vi "p09.vi"() -> ()   [LabVIEW 2015]
uses:
  <vilib>/regexp/Match Regular Expression.xnode
panel:
  out "Spreadsheet string -> array":dbl[][](array[numeric])
  out "Array -> spreadsheet string":string
  in  "time stamp":timestamp
  out "date/time string":string
  out "Scan - 2":string
  out "Scan -1":string
  out "remaining string":string
  out "X":dbl
  out "Y":i32
  out "Remaining String":string
  out "Unsigned Byte array to String":string
  out "String to Unsigned Byte array":u8[](array[numeric])
  out "String to Path":path
  out "Path to String":string
  out "Array to Path":path
  out "Path to Array":string[](array[string])
  out "offset past match":i32
  out "after match":string
  out "whole match":string
  out "before match":string
  out "offset past replacement":i32
  out "number of replacements":i32
  out "result string":string
  out "replaced substring":string
  out "result string":string
  out "string substring":string
  out "resulting string":string
  out "offset of match":i32
  out "match + rest of string":string
  out "substring before match":string
  out "offset past match":i32
  out "after substring":string
  out "match substring":string
  out "before substring":string
  out "Append String":string
  out "float-10 digit-2 decimal\n\"0\" padding":string
  out "binary-4 digit-\"0\"":string
  out "binary-4 digit-\" \"":string
  out "binary-without padding":string
  out "concatenated string":string
  out "Array":string[](array[string])
  out "CR & LF":string
  out "Double line feed":string
  out "Remainder":i32
  out "Quotient":i32
  out "Quotient":i32[](array[numeric])
  out "Remainder":i32[](array[numeric])
  out "Shift register":dbl[](array[numeric])
  out "Tunnel":dbl[](array[numeric])
  out "Final":dbl[](array[numeric])
  out "not of I16":i16
  out "not of U8":u8
  out "word swapped":i32 format="%032b"
  out "byte swapped":u32 format="%032b"
  out "?":dynamicdata(graph)
  out "number in bool":bool[](array[boolean])
  out "bool in number":dbl[](array[numeric])
  out "bool":bool[](array[boolean])
  out "number":dbl[](array[numeric])
  # "EXAMPLE - 1"
  # "EXAMPLE - 3"
  # "PATH / ARRAY FUNCTION"
  # "EXAMPLE - 2"
  # "APPEND T/F STRING"
  # "REPLACE SUBSTRING"
  # "MATCH REGULAR EXPRESSION"
  # "SCAN FROM STRING"
  # "ARRAY <-> SPREADSHEET\n STRING"
  # "EXAMPLE - 5"
  # "EXAMPLE - 4"
  # "EXAMPLE - 6"
  # "EXAMPLE - 7"
  # "FORMAT INTO STRING"
  # "SEARCH / SPLIT STRING"
  # "STRING SUBSET FUNCTION"
  # "MATCH PATTERN"
  # "STRING SUBSET FUNCTION"
  # "FORMAT DATE/TIME STRING"
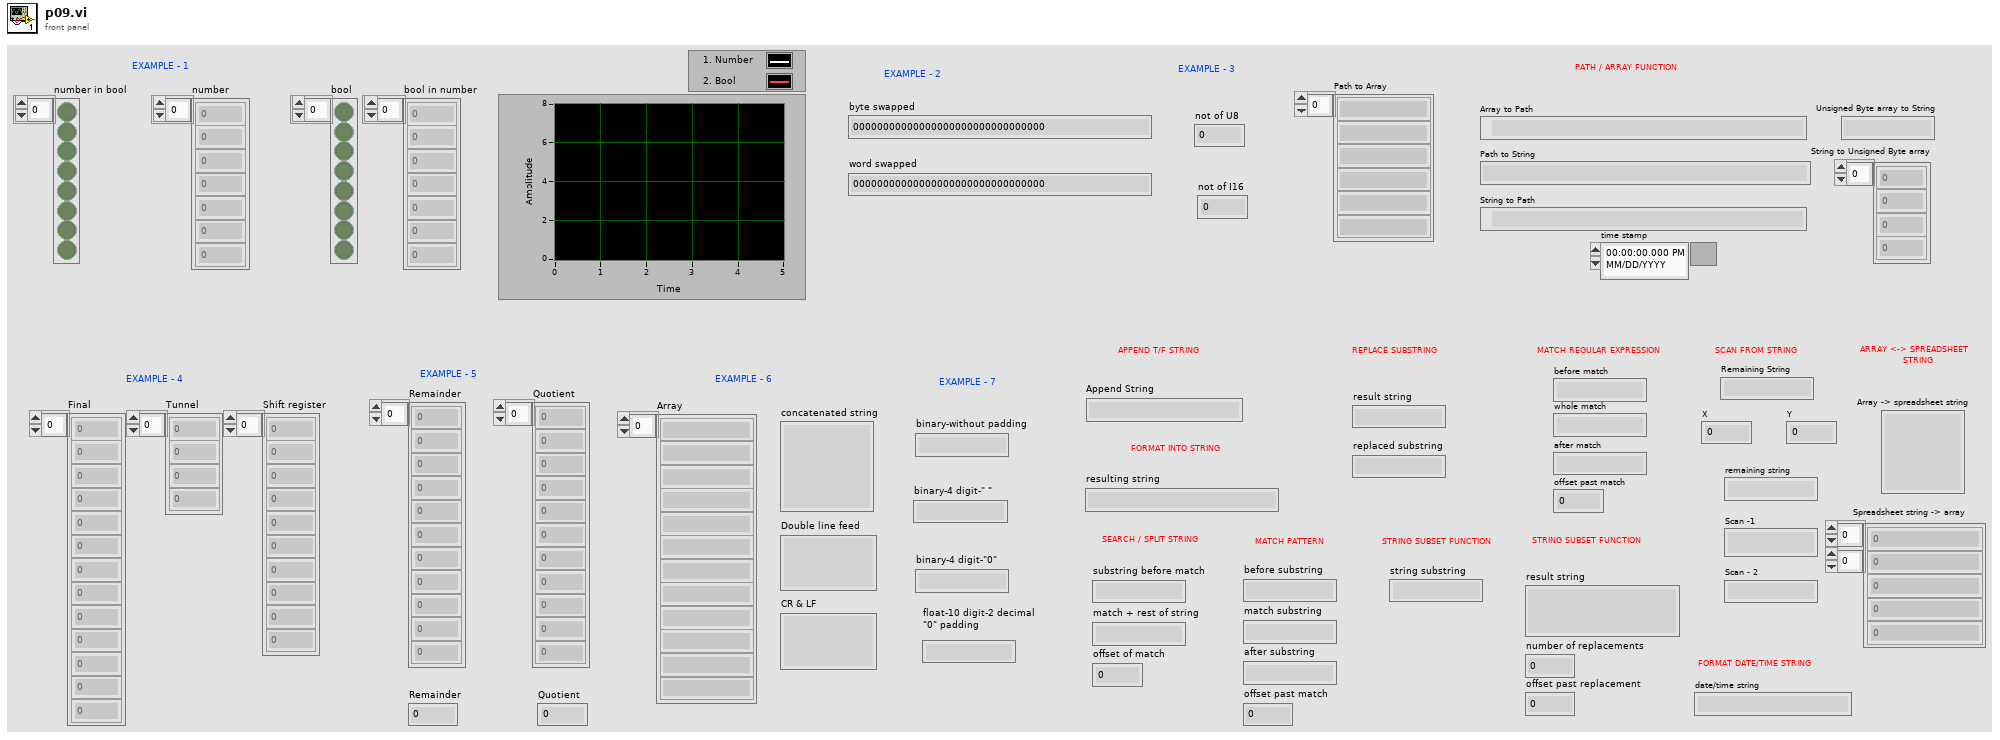
[diagram p1: front panel]
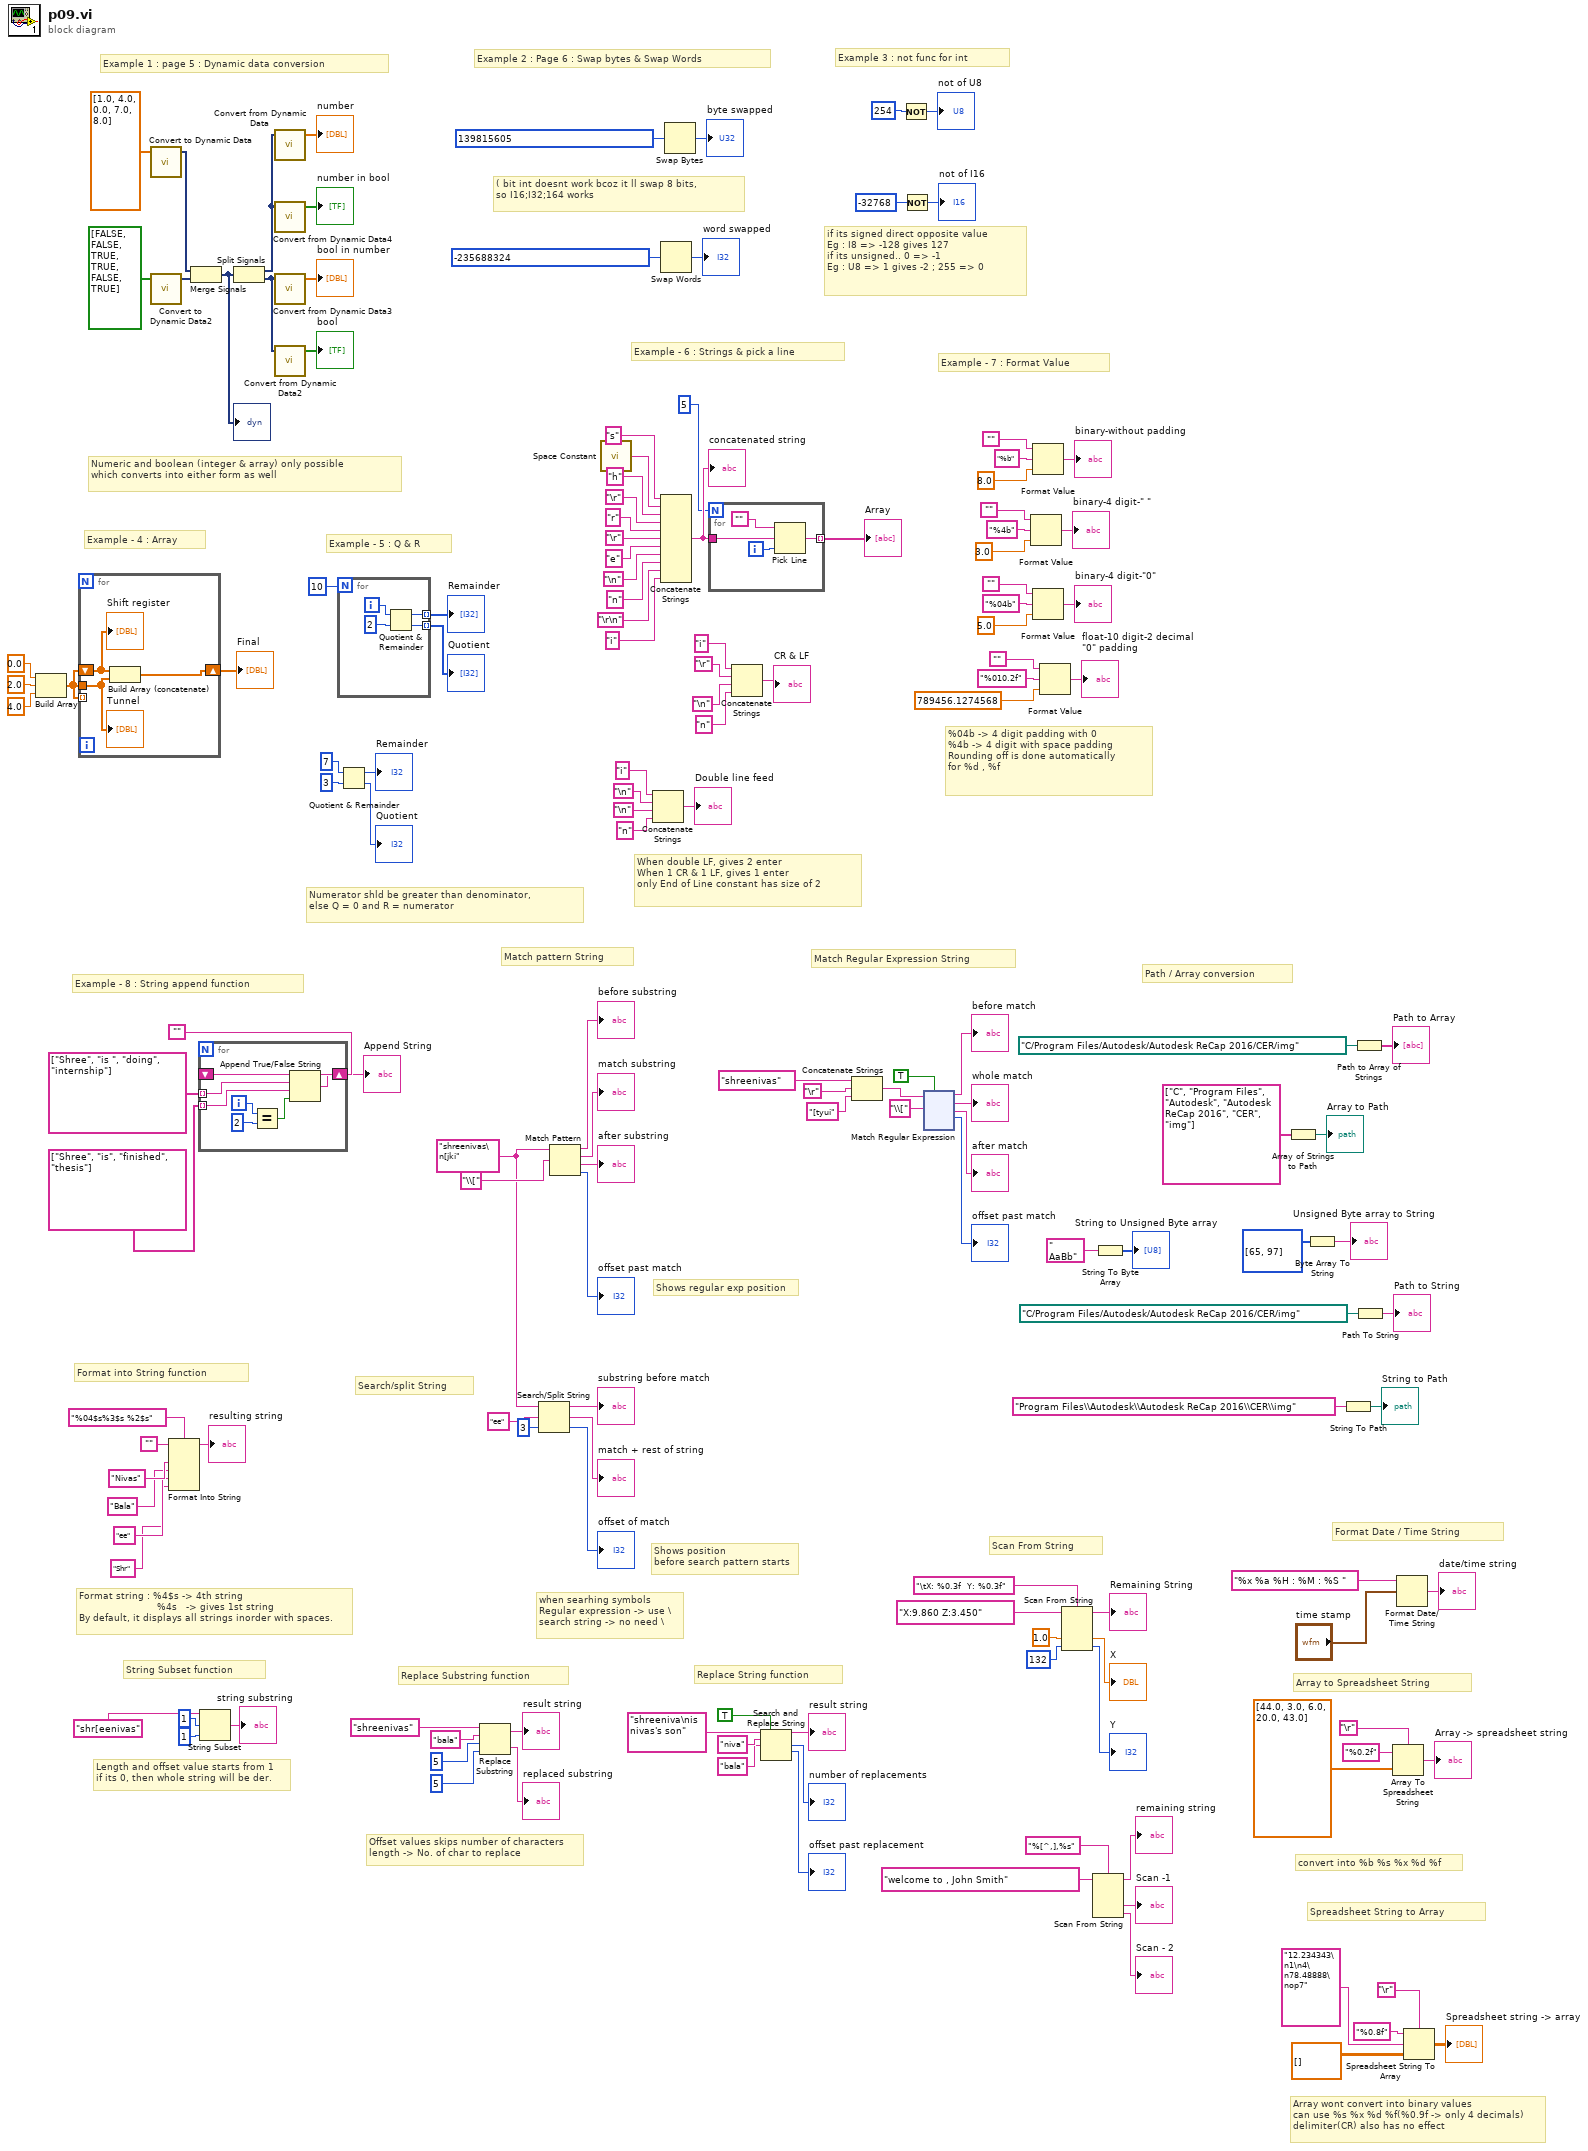
[diagram p0: block diagram]
diagram:
  w41 = "shreenivas\n[jki" ("string")
  # "Spreadsheet String to Array"
  # "convert into %b %s %x %d %f"
  # "Array wont convert into binary values\ncan use %s %x %d %f(%0.9f -> only 4 decimals)\ndelimiter(CR) also has no effect"
  # "Array to Spreadsheet String"
  # "Format Date / Time String"
  # "Scan From String"
  # "Path / Array conversion"
  # "Match Regular Expression String"
  # "Search/split String"
  # "Match pattern String"
  # "Offset values skips number of characters\nlength -> No. of char to replace"
  # "Replace String function"
  # "Replace Substring function"
  # "Shows position \nbefore search pattern starts"
  # "Shows regular exp position"
  # "when searhing symbols\nRegular expression -> use \\\nsearch string -> no need \\"
  # "Format string : %4$s -> 4th string\n                          %4s   -> gives 1st string\nBy default, it displays all strings inorder with spaces."
  # "Length and offset value starts from 1\nif its 0, then whole string will be der."
  # "Format into String function"
  # "String Subset function"
  # "Example - 8 : String append function"
  # "%04b -> 4 digit padding with 0\n%4b -> 4 digit with space padding\nRounding off is done automatically\nfor %d , %f"
  # "Example - 7 : Format Value"
  # "Example - 6 : Strings & pick a line"
  # "When double LF, gives 2 enter\nWhen 1 CR & 1 LF, gives 1 enter\nonly End of Line constant has size of 2"
  # "Numerator shld be greater than denominator, \nelse Q = 0 and R = numerator"
  # "Example - 5 : Q & R"
  # "Example - 4 : Array"
  # "if its signed direct opposite value \nEg : I8 => -128 gives 127\nif its unsigned.. 0 => -1\nEg : U8 => 1 gives -2 ; 255 => 0"
  # "Example 3 : not func for int"
  # "( bit int doesnt work bcoz it ll swap 8 bits, \nso I16;I32;164 works"
  # "Example 2 : Page 6 : Swap bytes & Swap Words"
  # "Numeric and boolean (integer & array) only possible\nwhich converts into either form as well"
  # "Example 1 : page 5 : Dynamic data conversion"
  n1 = Build Array(0.0 ("element"), 2.0 ("element"), 4.0 ("element")) -> (w134:dbl[])
  n2 = for {
    shift-right: [w158] -> w133
    shift-left: w134 -> [w157]
    tunnel: w134 -> [w159]
    tunnel: w134 -> [_] mode=indexing
    n3 = Build Array (concatenate)(w157, w159) -> (w158:dbl[])
    "Tunnel" <- w159
    "Shift register" <- w157
  }
  "Final" <- w133
  n4 = call "Convert to Dynamic Data"("Array"=dbl[] [1.0, 4.0, 0.0, 7.0, 8.0]) -> ("Dynamic Data Type"=w153:dynamicdata)  [unwired: 3 in]
  n5 = call "Convert to Dynamic Data2"("Array"=bool[] [FALSE, FALSE, TRUE, TRUE, FALSE, TRUE]) -> ("Dynamic Data Type"=w154:dynamicdata)  [unwired: 3 in]
  n6 = Format Into String(format string="%04$s%3$s %2$s", initial string="", "Nivas" ("initial string"), "Bala" ("initial string"), "ee" ("initial string"), "Shr" ("initial string")) -> (resulting string=→"resulting string":string)  [unwired: 1 in, 1 out]
  n7 = Merge Signals(w153, w154) -> (w152:dynamicdata)
  "?" <- w152
  n8 = for {
    tunnel: string[] ["Shree", "is ", "doing", "internship"] -> [w166] mode=indexing
    tunnel: string[] ["Shree", "is", "finished", "thesis"] -> [w165] mode=indexing
    shift-right: [w160] -> w83
    shift-left: "" -> [w161]
    i -> [w164]
    n9 = Equal?(x=w164, y=2) -> (x = y?=w162:bool)
    n10 = Append True/False String(1:w162, 2:w165, 3:w166, 4:w161) -> (0:w160:string)
  }
  "Append String" <- w83
  n11 = String Subset(string="shr[eenivas", offset (0)=1, length (rest)=1 ("length (rest)")) -> (substring=→"string substring":string)
  n12 = Split Signals(w152) -> (w146:dynamicdata, w148:dynamicdata)  [unwired: 2 in]
  n13 = call "Convert from Dynamic Data"("Dynamic Data Type"=w146) -> ("Array"=→"number":dbl[])  [unwired: 3 in]
  n14 = call "Convert from Dynamic Data4"("Dynamic Data Type"=w146) -> ("Array"=→"number in bool":bool[])  [unwired: 3 in]
  n15 = call "Convert from Dynamic Data3"("Dynamic Data Type"=w148) -> ("Array"=→"bool in number":dbl[])  [unwired: 3 in]
  n16 = call "Convert from Dynamic Data2"("Dynamic Data Type"=w148) -> ("Array"=→"bool":bool[])  [unwired: 3 in]
  n17 = for {
    N: 10 -> [_]
    tunnel: [w168] -> w131 mode=indexing
    tunnel: [w167] -> w130 mode=indexing
    i -> [w170]
    n18 = Quotient & Remainder(x=w170, y=2) -> (x-y*floor(x/y)=w168:i32, floor(x/y)=w167:i32)
  }
  "Remainder" <- w131
  "Quotient" <- w130
  n19 = Quotient & Remainder(x=7 ("y"), y=3) -> (x-y*floor(x/y)=→"Remainder":i32, floor(x/y)=→"Quotient":i32)
  n20 = Replace Substring(2:5 ("length (len. of substring)"), 3:5 ("offset (0)"), 4:"bala" ("substring (\"\")"), 5:"shreenivas" ("string")) -> (0:→"replaced substring":string, 1:→"result string":string)
  n21 = Search/Split String(string=w41, search string/char (-)="ee" ("string"), offset (0)=3) -> (substring before match=→"substring before match":string, match + rest of string=→"match + rest of string":string, offset of match=→"offset of match":i32)
  n22 = Match Pattern(string=w41, regular expression="\\[" ("string")) -> (before substring=→"before substring":string, match substring=→"match substring":string, after substring=→"after substring":string, offset past match=→"offset past match":i32)  [unwired: 1 in]
  n23 = call <vilib>:"Space Constant.vi"() -> ("String"=w124:string)
  n24 = Concatenate Strings("i", "\n", "\n", "n") -> (→"Double line feed":string)
  n25 = Swap Words(1:-235688324) -> (0:→"word swapped":i32)
  n26 = Concatenate Strings("s", w124, "h", "\r", "r", "\r", "e", "\n", "n", "\r\n", "i") -> (w104:string)
  "concatenated string" <- w104
  n27 = Swap Bytes(anything=u32 139815605 ("data")) -> (byte swapped=→"byte swapped":u32)
  n28 = for {
    N: 5 -> [_]
    tunnel: w104 -> [w172]
    tunnel: [w173] -> w102 mode=indexing
    i -> [w174]
    n29 = Pick Line(string ("")="", multi-line string=w172, line index=w174) -> (output string=w173:string)
  }
  "Array" <- w102
  n30 = Concatenate Strings("i", "\r", "\n", "n") -> (→"CR & LF":string)
  n31 = Search and Replace String(replace all?=TRUE ("replace all? (F)"), input string="shreeniva\nis nivas's son" ("string"), search string="niva" ("substring (\"\")"), replace string="bala" ("substring (\"\")")) -> (result string=→"result string":string, number of replacements=→"number of replacements":i32, offset past replacement=→"offset past replacement":i32)  [unwired: 4 in, 1 out]
  n32 = Concatenate Strings("shreenivas" ("string"), "\r", "[tyui" ("string")) -> (w37:string)
  n33 = Not(x=u8 254) -> (.not. x?=→"not of U8":u8)
  n34 = Not(x=i16 -32768) -> (.not. x?=→"not of I16":i16)
  n35 = xnode "Match Regular Expression"("input string"=w37, "regular expression"="\\[", "ignore case? (F)"=TRUE) -> ("before match"=→"before match":string, "whole match"=→"whole match":string, "after match"=→"after match":string, "offset past match"=→"offset past match":i32)  [unwired: 3 in, 1 out]
  n36 = Format Value(string ("")="", format string="%4b", value (0)=3.0) -> (output string=→"binary-4 digit-\" \"":string)
  n37 = Format Value(string ("")="", format string="%b", value (0)=8.0) -> (output string=→"binary-without padding":string)
  n38 = Format Value(string ("")="", format string="%04b", value (0)=5.0) -> (output string=→"binary-4 digit-\"0\"":string)
  n39 = Format Value(string ("")="", format string="%010.2f", value (0)=789456.1274568) -> (output string=→"float-10 digit-2 decimal\n\"0\" padding":string)
  n40 = Scan From String(format string="\tX: %0.3f  Y: %0.3f", input string="X:9.860 Z:3.450" ("string"), default 1=1.0 ("default value 1"), default 2=132 ("default value 1")) -> (remaining string=→"Remaining String":string, output 1=→"X":dbl, output 2=→"Y":i32)  [unwired: 2 in, 2 out]
  n41 = Scan From String(format string="%[^,],%s", input string="welcome to , John Smith" ("string")) -> (remaining string=→"remaining string":string, output 1=→"Scan -1":string, output 2=→"Scan - 2":string)  [unwired: 4 in, 2 out]
  n42 = String To Byte Array(string="  AaBb" ("Path to String 2")) -> (unsigned byte array=→"String to Unsigned Byte array":u8[])
  n43 = Array of Strings to Path(0:string[] ["C", "Program Files", "Autodesk", "Autodesk ReCap 2016", "CER", "img"] ("array of strings 2")) -> (2:→"Array to Path":path)  [unwired: 1 in]
  n44 = Byte Array To String(unsigned byte array=u8[] [65, 97]) -> (string=→"Unsigned Byte array to String":string)
  n45 = String To Path(string="Program Files\\Autodesk\\Autodesk ReCap 2016\\CER\\img" ("Path to String 2")) -> (path=→"String to Path":path)
  n46 = Path to Array of Strings(0:path "C:/Program Files/Autodesk/Autodesk ReCap 2016/CER/img" ("path")) -> (2:→"Path to Array":string[])  [unwired: 1 out]
  n47 = Path To String(path=path "C:/Program Files/Autodesk/Autodesk ReCap 2016/CER/img") -> (string=→"Path to String":string)
  n48 = Array To Spreadsheet String(delimiter (Tab)="\r", array=dbl[] [44.0, 3.0, 6.0, 20.0, 43.0], 3:"%0.2f" ("format string")) -> (spreadsheet string=→"Array -> spreadsheet string":string)
  n49 = Format Date/Time String(time format string (%c)="%x %a %H : %M : %S ", seconds (now)="time stamp") -> (date/time string=→"date/time string":string)  [unwired: 1 in]
  n50 = Spreadsheet String To Array(delimiter (Tab)="\r", format string="%0.8f", spreadsheet string="12.234343\n1\n4\n78.48888\nop7" ("spreadsheet string 2"), array type (2D Dbl)=dbl[][] []) -> (array=→"Spreadsheet string -> array":dbl[][])
